vi "未命名 1.vi"() -> ()   [LabVIEW 2011, in "迭代器.lvlib"]
panel:
  out "年龄":u8
  out "姓名":string
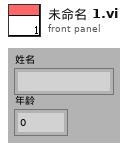
[diagram p1: front panel]
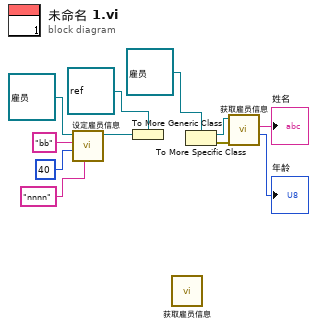
[diagram p0: block diagram]
diagram:
  n1 = call "设定雇员信息.vi"("职务"="nnnn", "年龄"=u8 40, "姓名"="bb", "雇员 输入"=refnum<class "雇员.lvclass"> refnum ("迭代器.lvlib:雇员.lvclass")) -> ("雇员 输出"=w8:refnum<class "雇员.lvclass">)  [unwired: 6 in, 1 out]
  n2 = To More Generic Class(target class=refnum<class> refnum ("LabVIEW对象"), reference=w8) -> ()  [unwired: 1 out]
  n3 = call-dynamic "获取雇员信息.vi"() -> ()  [unwired: 7 in, 5 out]
  n4 = To More Specific Class(target class=refnum<class "雇员.lvclass"> refnum ("迭代器.lvlib:雇员.lvclass")) -> (specific class reference=w5:refnum<class "雇员.lvclass">, error out=w4:errorcluster)  [unwired: 2 in]
  n5 = call-dynamic "获取雇员信息.vi"("error in (no error)"=w4, "雇员 输入"=w5) -> ("年龄"=→"年龄":u8, "姓名"=→"姓名":string)  [unwired: 5 in, 3 out]
